vi "comm read.vi"(8 "error in (no error)":errorcluster, 10 "requested byte count":u32, 11 "Comm Handle":u32) -> (0 "error out":errorcluster, 1 "byte count":u32, 2 "string read":string, 3 "dup Comm Handle":u32)   [LabVIEW 2013, in "lvserial.lvlib"]
doc: "Reads bytes from the serial port and stores the data into the specified buffer."
uses:
  lvserial.lvlib
  lvserial.dll
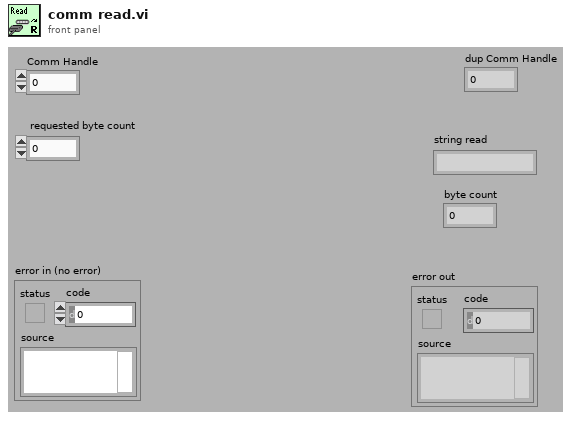
[diagram p1: front panel]
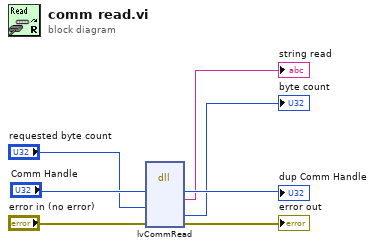
[diagram p0: block diagram]
diagram:
  n1 = dll-call lib="lvserial.dll" fn="lvCommRead"("hComm"="Comm Handle", "ulBytesToRead"="requested byte count", "error in (no error)"="error in (no error)") -> ("hComm"=→"dup Comm Handle":u32, "Buffer"=→"string read":string, "pulBytesRead"=→"byte count":u32, "error in (no error)"=→"error out":errorcluster)  [unwired: 5 in, 4 out]
